vi "close.vi"(8 "error in (no error)":errorcluster, 11 "Keithley2002 in":refnum<class "Keithley2002.lvclass">) -> (0 "error out":errorcluster, 3 "Keithley2002 out":refnum<class "Keithley2002.lvclass">)   [LabVIEW 2019, in "Keithley2002.lvclass"]
uses:
  Keithley2002.lvclass
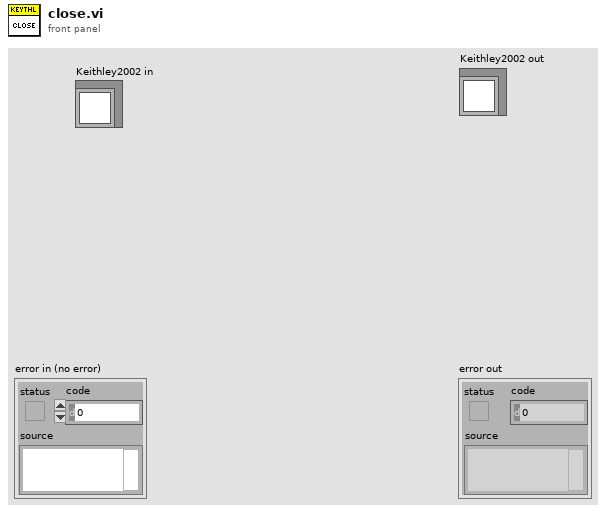
[diagram p1: front panel]
types:
  T1 = cluster{"error":bool, "code":i32, "source":string}
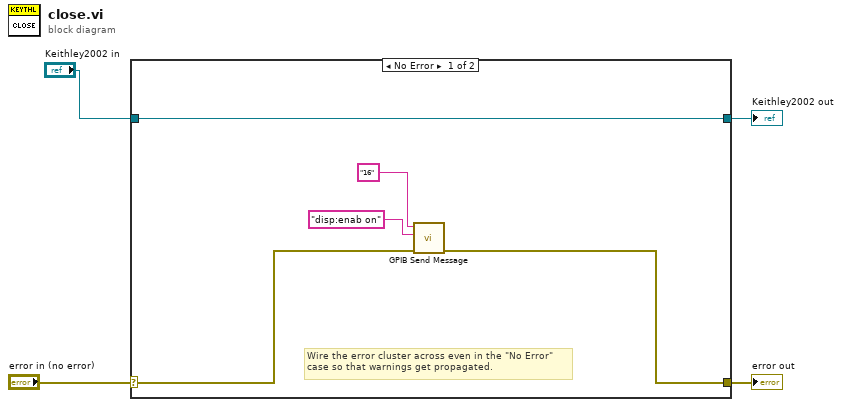
[diagram p0: block diagram]
diagram:
  n1 = case shown="No Error" "error in (no error)" {
    selector: "error in (no error)" -> [w6 w11]
    tunnel: [w5 w11] -> w3
    tunnel: [w9 w10] -> w1
    tunnel: "Keithley2002 in" -> [w9 w10]
    frame No Error {
      # "Wire the error cluster across even in the \"No Error\"\ncase so that warnings get propagated."
      n2 = call <instrlib>:"GPIB Send Message.vi"("address string"="16" ("write buffer"), "write buffer"="disp:enab on", "error in"=w6) -> ("error out"=w5:T1)  [unwired: 4 in, 2 out]
    }
    frame Error {
    }
  }
  "error out" <- w3
  "Keithley2002 out" <- w1
